vi "Process Data.vi"(8 "error in":errorcluster, 11 "Simple Client with Async Process in":refnum<class "Simple Client with Async Process.lvclass">) -> (0 "error out":errorcluster, 3 "Simple Client with Async Process out":refnum<class "Simple Client with Async Process.lvclass">)   [LabVIEW 2014, in "Simple Client with Async Process.lvclass"]
uses:
  Simple Client with Async Process.lvclass
  Architecture/Classes/Topic_class/Topic.lvclass
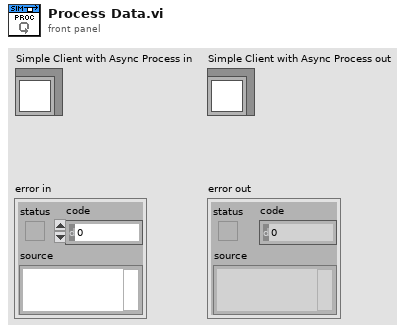
[diagram p1: front panel]
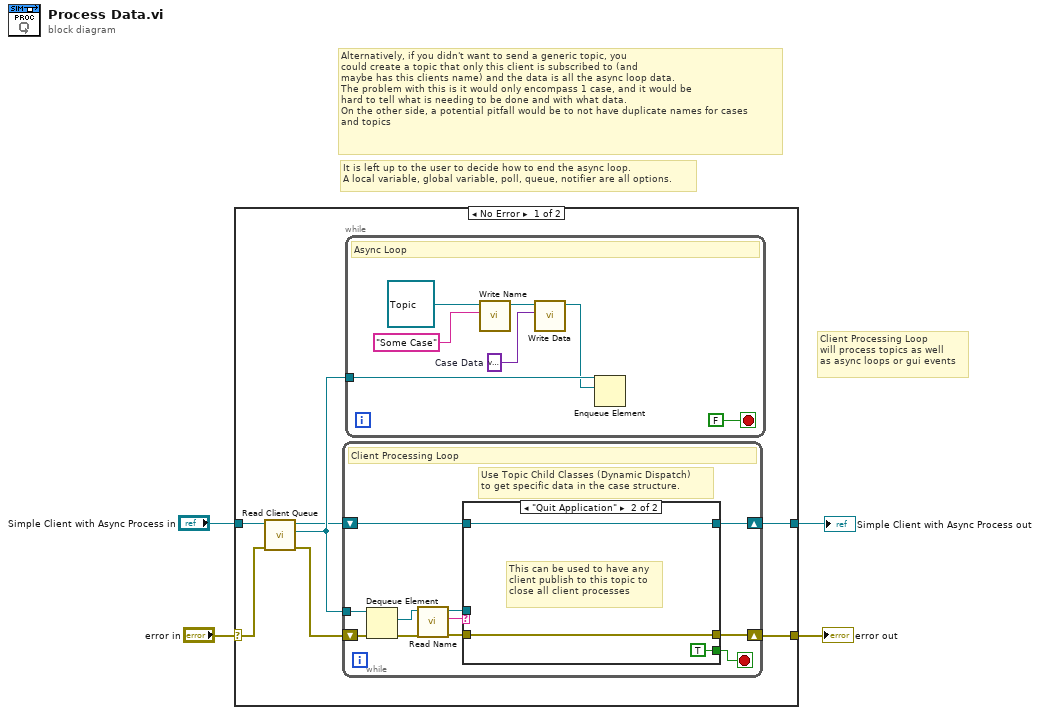
[diagram p0: block diagram]
diagram:
  # "It is left up to the user to decide how to end the async loop.  \nA local variable, global variable, poll, queue, notifier are all options."
  # "Alternatively, if you didn't want to send a generic topic, you\ncould create a topic that only this client is subscribed to (and\nmaybe has this clients name) and the data is all the async loop data.\nThe problem with this is it would only encompass 1 case, and it would be \nhard to tell what is needing to be done and with what data.\nOn the other side, a potential pitfall would be to not have duplicate names for cases\nand topics"
  # "Client Processing Loop\nwill process topics as well\nas async loops or gui events"
  n1 = case shown="No Error" "error in" {
    selector: "error in" -> [w8 w36]
    tunnel: [w9 w36] -> w1
    tunnel: [w5 w35] -> w3
    tunnel: "Simple Client with Async Process in" -> [w11 w35]
    frame No Error {
      n2 = call-dynamic "Read Client Queue.vi"("error in"=w8, "Client in"=w11) -> ("error out"=w10:errorcluster, "Client Queue"=w7:refnum<queue>, "Client out"=w6:refnum<class "Simple Client with Async Process.lvclass">)  [unwired: 7 in]
      n3 = while {
        tunnel: w7 -> [w29]
        shift-right: [w21] -> w9
        shift-left: w10 -> [w22]
        shift-right: [w19] -> w5
        shift-left: w6 -> [w20]
        stop <- w23 stop-if-true
        # "Use Topic Child Classes (Dynamic Dispatch)\nto get specific data in the case structure."
        # "Client Processing Loop"
        n4 = Dequeue Element(queue=w29, error in (no error)=w22) -> (element=w27:refnum<class "Topic.lvclass">, error out=w28:errorcluster)  [unwired: 1 in, 2 out]
        n5 = call-dynamic "Read Name.vi"("error in"=w28, "Topic in"=w27) -> ("error out"=w25:errorcluster, "Name"=w26:string, "Topic out"=w24:refnum<class "Topic.lvclass">)  [unwired: 7 in]
        n6 = case shown="\"Quit Application\"" w26 {
          tunnel: [_ TRUE] -> w23
          tunnel: w25 -> [w31 w33]
          tunnel: [w31 w33] -> w21
          tunnel: w24 -> [_ _]
          tunnel: w20 -> [w30 w32]
          tunnel: [w30 w32] -> w19
          frame Default {
          }
          frame "Quit Application" {
            # "This can be used to have any\nclient publish to this topic to\nclose all client processes"
          }
        }
      }
      n7 = while {
        tunnel: w7 -> [w18]
        stop <- FALSE stop-if-true
        w14 = variant  # Case Data
        # "Async Loop"
        n8 = call-dynamic "Write Name.vi"("Name"="Some Case", "Topic in"=refnum<class "Topic.lvclass"> refnum ("Topic.lvclass")) -> ("Topic out"=w15:refnum<class "Topic.lvclass">)  [unwired: 8 in, 1 out]
        n9 = call-dynamic "Write Data.vi"("Data"=w14, "Topic in"=w15) -> ("Topic out"=w13:refnum<class "Topic.lvclass">)  [unwired: 8 in, 1 out]
        n10 = Enqueue Element(queue=w18, element=w13) -> ()  [unwired: 2 in, 3 out]
      }
    }
    frame Error {
    }
  }
  "error out" <- w1
  "Simple Client with Async Process out" <- w3
